vi "NextStep.vi"(8 "error in":errorcluster, 10 "E-CD+ STEPS":T1=enum."01 - Engage Clamp" caption="Next:", 11 "Enum in":refnum<vi>) -> (0 "error out":errorcluster)   [LabVIEW 2016]
uses:
  Controls/E-CD+ State.ctl
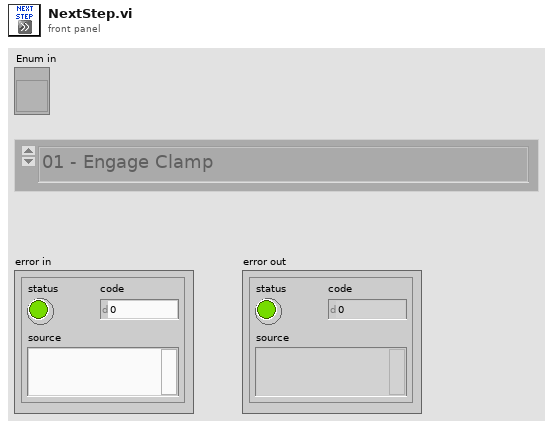
[diagram p1: front panel]
types:
  T1 = typedef "E-CD+ State.ctl" = enum16{"00 - Stop", "01 - Engage Clamp", "02 - Drive BR Left to Align TWT", "03 - Drive TWT Forward", "04 - Rotate OT CW to Engage", "05 - Rotate IT CCW to Engage", "06 - Rotate IT CCW to Disengage Bleeder Valve", "07 - Leak Detection", "08 - Remove Safety Plug", "09 - Drive BR Right to Align DL", "10 - Drive DL Forward", "11 - Install DL", "12 - Continuous Circulation", "13 - Remove DL", "14 - Drive DL Backward for Cleaning", "15 - Clean Camera and Threads", "16 - Drive DL Backward", "17 - Drive BR Left to Align TWT", "18 - Install Safety Plug", "19 - Install Bleeder Valve", "20 - Drive TWT Backward", "21 - Drive BR Right to Initial Position"}
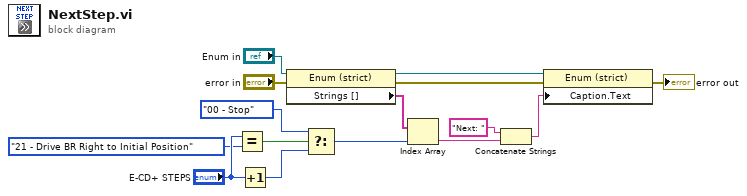
[diagram p0: block diagram]
diagram:
  n1 = Equal?(x="E-CD+ STEPS", y=E-CD+_State."21 - Drive BR Right to Initial Position" ("E-CD+ STEPS")) -> (x = y?=w4:bool)
  n2 = Increment(x="E-CD+ STEPS") -> (x+1=w2:T1)
  n3 = property on="Property Node" class="Enum (strict)"(reference="Enum in", error in="error in") -> (reference out=w15:refnum<vi>, error out=w13:errorcluster, "Strings []"=w8:string[])
  n4 = Select(t=E-CD+_State."00 - Stop" ("E-CD+ STEPS"), s=w4, f=w2) -> (s? t:f=w1:T1)
  n5 = Index Array(array=w8, index=w1) -> (element=w10:string)
  n6 = Concatenate Strings("Next: " ("string"), w10) -> (w11:string)
  n7 = property on="Property Node" class="Enum (strict)"(reference=w15, error in=w13, "Caption.Text"=w11) -> (error out=→"error out":errorcluster)  [unwired: 1 out]
